vi "VRM Spherical to Cartesian.vi"(8 "error in (no error)":errorcluster, 11 "Field (r,theta,phi)":dbl[](array[numeric])) -> (0 "error out":errorcluster, 3 "Field (x,y,z)":dbl[](array[numeric]))   [LabVIEW 2019, in "Instrument.OxfordVRM.lvclass"]
uses:
  Instrument.OxfordVRM.lvclass
  <vilib>/Analysis/coordinate.llb/3D Coordinate Conversion (Scalar).vi
  <vilib>/Analysis/NI_AALPro.lvlib
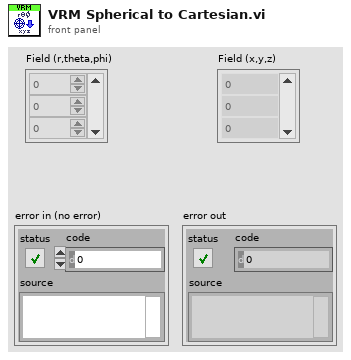
[diagram p1: front panel]
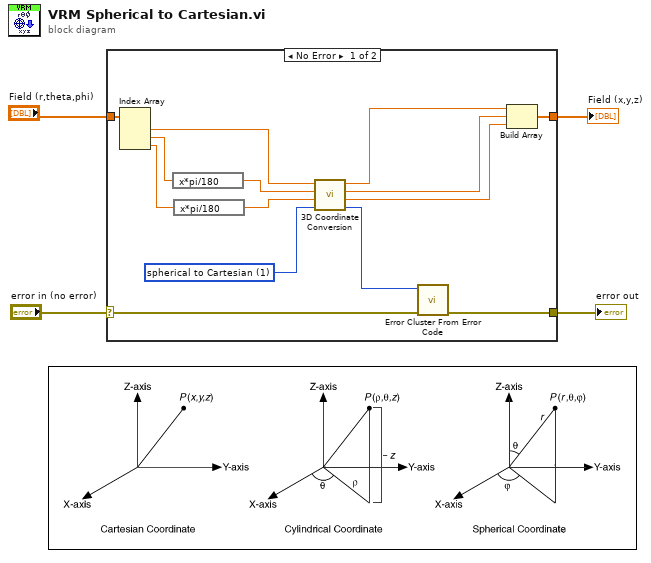
[diagram p0: block diagram]
diagram:
  n1 = case shown="No Error" "error in (no error)" {
    selector: "error in (no error)" -> [w16 w19]
    tunnel: [w15 w19] -> w3
    tunnel: "Field (r,theta,phi)" -> [w14 _]
    tunnel: [w12 _] -> w1
    frame No Error {
      w18 = u16 1 items=["Cartesian to spherical", "spherical to Cartesian", "Cartesian to cylindrical", "cylindrical to Cartesian", "spherical to cylindrical", "cylindrical to spherical"] ("conversion type")
      n2 = Index Array(array=w14) -> (element #1=w9:dbl, element #2=w11:dbl, element #3=w8:dbl)  [unwired: 3 in]
      n3 = expression code="x*pi/180"(w11) -> (w10:dbl)
      n4 = expression code="x*pi/180"(w8) -> (w7:dbl)
      n5 = call-poly <vilib>:"3D Coordinate Conversion.vi"("conversion type"=w18, "axis 3"=w7, "axis 2"=w10, "axis 1"=w9) -> ("error"=w17:i32, "axis 3 out"=w5:dbl, "axis 2 out"=w6:dbl, "axis 1 out"=w13:dbl)  [unwired: 4 in]
      n6 = call <vilib>:"Error Cluster From Error Code.vi"("error in (no error)"=w16, "error code (0)"=w17) -> ("error out"=w15:errorcluster)  [unwired: 7 in]
      n7 = Build Array(w13, w6, w5) -> (w12:dbl[])
    }
    frame Error {
    }
  }
  "error out" <- w3
  "Field (x,y,z)" <- w1
